vi "Run VI Without Panel.vi"(8 "error in":errorcluster, 11 "VI Reference":refnum<vi>) -> (0 "error out":errorcluster, 3 "vi reference":refnum<vi>)   [LabVIEW 2015]
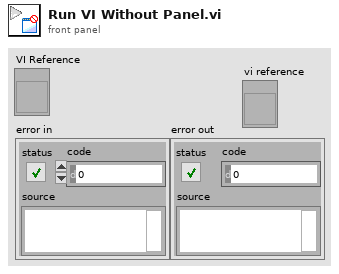
[diagram p1: front panel]
types:
  T1 = enum32{"Bad", "Idle", "Run top level", "Running"}
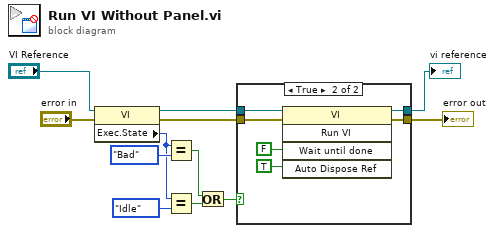
[diagram p0: block diagram]
diagram:
  n1 = property class="VI"(reference="VI Reference", error in="error in") -> (reference out=w9:refnum<vi>, error out=w8:errorcluster, "Exec.State"=w1:T1)
  n2 = Equal?(x=w1, y=T1."Bad" ("Execution:State")) -> (x = y?=w10:bool)
  n3 = Equal?(x=w1, y=T1."Idle" ("Execution:State")) -> (x = y?=w2:bool)
  n4 = Or(x=w10, y=w2) -> (x .or. y?=w5:bool)
  n5 = case shown="True" w5 {
    tunnel: w9 -> [w13 w17]
    tunnel: w8 -> [w14 w16]
    tunnel: [w14 w19] -> w7
    tunnel: [w13 w15] -> w6
    frame False {
    }
    frame True {
      n6 = invoke class="VI" method="Run VI"(reference=w17, error in=w16, "Wait until done"=FALSE ("Wait Until Done"), "Auto Dispose Ref"=TRUE ("Auto Dispose Reference")) -> (reference out=w15:refnum<vi>, error out=w19:errorcluster)  [unwired: 1 in, 3 out]
    }
  }
  "error out" <- w7
  "vi reference" <- w6
